vi "FPGA_Main_IX.vi"() -> ()   [LabVIEW 2018]
uses:
  <vilib>/LabVIEW Targets/FPGA/RIO/BlueMoonOnboardIO/nicrio_cRIO-BlueMoonOnboardAi_TerminalMod.ctl
  <vilib>/LabVIEW Targets/FPGA/RIO/BlueMoonOnboardIO/nicrio_cRIO-BlueMoonOnboardAi_VoltageRange.ctl
  <vilib>/Platform/TimedLoop/XDataNode/timing_clust.ctl
  <vilib>/Platform/TimedLoop/XDataNode/nitl_modes.ctl
  <vilib>/Platform/TimedLoop/XDataNode/wakeup.ctl
  ctl/_FPGA_priRFSettings_Parameters.ctl
  ctl/_FPGA_auxWfmSettings_Parameters.ctl
  <vilib>/rvi/Emulation/niFpgaGetClockAttributes.vi
  <vilib>/rvi/Emulation/niFpgaSctlEmulationGetInTimedLoop.vi
  <vilib>/rvi/Emulation/niFpgaEmulationReportErrorSimple.vi
  <vilib>/rvi/Emulation/niFpgaEmulationIsFPGAContextNoSignature.vi
  <vilib>/rvi/DataTransferAndStorage/Container/Common/niFpgaContainerGetUniqueNameForEmu.vi
  <vilib>/rvi/Memory/Memory_Emulation/niFpgaMemoryEmulationCacheClearOnFirstRun.vi
  <vilib>/rvi/Memory/Memory_Emulation/nirvimemoryEmulationManagerCache_MakeExclusive.vi
  <vilib>/rvi/Memory/Memory_Emulation/niFpgaMemoryEmulationValidateCache.vi
  <vilib>/rvi/Memory/Memory_Emulation/nirvimemoryEmulationManagerCache_InsertValue.vi
  <vilib>/Utility/error.llb/Clear Errors.vi
  <vilib>/rvi/Memory/Memory_Emulation/nirvimemoryEmulationManagerCache_ReleaseExclusive.vi
  <vilib>/rvi/Memory/Memory_Emulation/nirvimemoryEmulationManagerCache_GetValue.vi
  <vilib>/rvi/Memory/Memory_Emulation/nirvimemoryEmulationManagerCache_SetValue.vi
  <vilib>/rvi/Emulation/niFpgaProcessEmulError.vi
  <vilib>/rvi/eio/common/nirviEmuTemplateMethod_errors.vi
  <vilib>/rvi/Emulation/niFpgaCriticalErrorInLSC.vi
  <vilib>/rvi/eio/common/nirviEmuTemplatePropertySet_noerrors.vi
  <vilib>/rvi/errors/niFpgaSetErrorForExecOnDevCompSimple.vi
  <vilib>/rvi/eio/common/nirviEmuReportErrorAndStop.vi
  <vilib>/rvi/FIFO/Fifo_Resource/nirvififoEmulationSetSize.vi
  <vilib>/rvi/FIFO/Fifo_Resource/nirviFifoEmulationQueueMgr.vi
  <instcachedir>/0/nirviFifoEmulationQueueMgr_E5CAEC123FF24DC58D834DCA3CDAA9B5.lvgen/nirviFifoEmulationQueueMgr_E5CAEC123FF24DC58D834DCA3CDAA9B5_004.vi
  <vilib>/rvi/FIFO/Fifo_Resource/nirvififoEmulationDetermineInputValidOut.vi
  <vilib>/rvi/FIFO/Fifo_Resource/nirvififoEmulationCreateLock.vi
  <vilib>/rvi/FIFO/Fifo_Resource/nirvififoEmulationObtainLock.vi
  <vilib>/rvi/FIFO/Fifo_Resource/nirvififoEmulationReleaseLock.vi
  <vilib>/rvi/occurrence/nirviWaitOnOccurrenceBase.vi
  <vilib>/rvi/errors/nirviReportUnexpectedCaseInternalError.vi
  <vilib>/rvi/errors/nirviReportUnexpectedCaseInternalError (U32).vi
  <instcachedir>/0/nirviFifoEmulationQueueMgr_E5CAEC123FF24DC58D834DCA3CDAA9B5.lvgen/nirviFifoEmulationQueueMgr_E5CAEC123FF24DC58D834DCA3CDAA9B5_006.vi
  <instcachedir>/0/nirviFifoEmulationQueueMgr_E5CAEC123FF24DC58D834DCA3CDAA9B5.lvgen/nirviFifoEmulationQueueMgr_E5CAEC123FF24DC58D834DCA3CDAA9B5_002.vi
  <instrlib>/_niInstr/Basic Elements/v1/FPGA/Private/Count Down U16.vi
  <instrlib>/_niInstr/Basic Elements/v1/FPGA/Private/Count Down U32.vi
  <vilib>/rvi/interface/RandomDataEmulation/niFpgaRandomDataHandleErrors.vi
  <instcachedir>/0/nirviFifoEmulationQueueMgr_E5CAEC123FF24DC58D834DCA3CDAA9B5.lvgen/nirviFifoEmulationQueueMgr_E5CAEC123FF24DC58D834DCA3CDAA9B5_003.vi
  <vilib>/rvi/Memory/Memory_Emulation/nirvimemoryFastEmulation.vi
  <vilib>/rvi/Memory/Memory_Emulation/nirvimemoryEmulation.vi
  <vilib>/rvi/DataTransferAndStorage/Container/XNode/niFpgaContainer.xnode
  <vilib>/rvi/DataTransferAndStorage/Register/Emulation/niFpgaRegisterEmulation.vi
  <vilib>/eio/EIONode/EIONode.xnode
  <vilib>/eio/EIOPropertyNode/EIOPropertyNode.xnode
  <vilib>/rvi/FIFO/Fifo_Resource/nirvififoEmulationWrite.vi
  <vilib>/Platform/TimedLoop/XDataNode/XDataNode.xnode
  <vilib>/rvi/FIFO/Fifo_Resource/nirvififoEmulationRead.vi
  <vilib>/rvi/interface/RandomDataEmulation/nirviRandomDataFpgaReadWriteTemplate.vi
  <vilib>/rvi/FXPMathLib/FxpAdd/XNode/nifxpmath_Add.xnode
  <instrlib>/_niInstr/Basic Elements/v1/FPGA/niInstr Basic Elements v1 FPGA.lvlib
  <vilib>/rvi/FXPMathLib/sim/FxpSim.dll
  <vilib>/Platform/TimedLoop/XDataNode/XDNodeRunTimeDep.lvlib
  <vilib>/rvi/eio/common/nirviEmuTemplatePropertyGet_errors.vi
  <vilib>/rvi/eio/common/nirviEmuTemplatePropertyGet_noerrors.vi
  <vilib>/rvi/eio/common/nirviEmuTemplatePropertySet_errors.vi
panel:
  out "DI":u8
  out "Daq.AqNumber?":u32
  out "Daq.HighestValue_I16":i16
  out "Daq.Length?":u32
  out "Act.Timeout":u16
  out "Aux.Timeout":u16
  out "Pri.Timeout":u16
  out "AI.ReadingClocks":u32
  in  "Action":bool
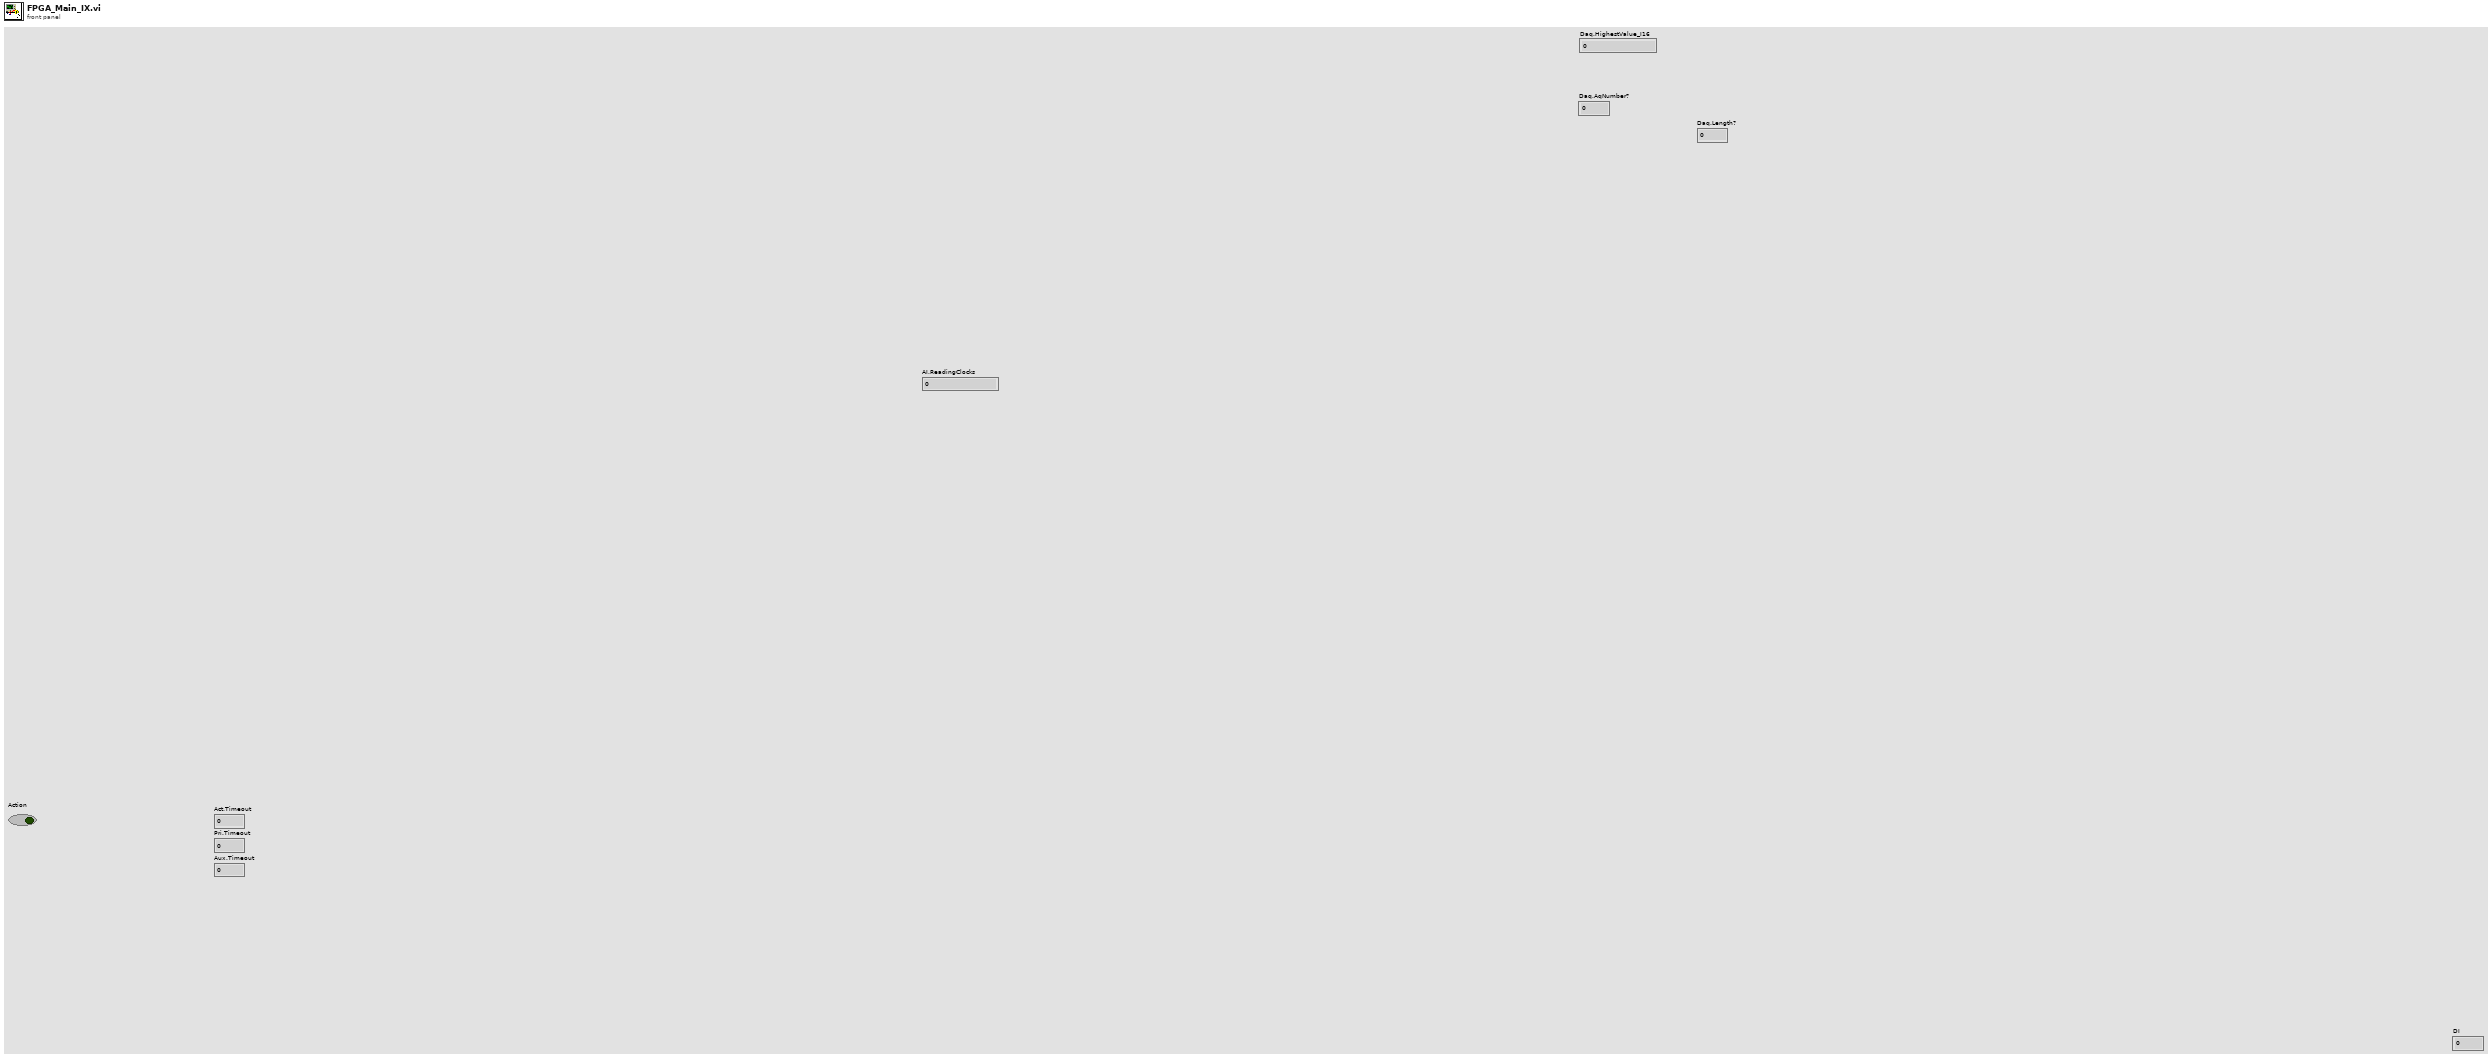
[diagram p1: front panel]
types:
  T1 = typedef "nicrio_cRIO-BlueMoonOnboardAi_VoltageRange.ctl" = u8
  T2 = typedef "nicrio_cRIO-BlueMoonOnboardAi_TerminalMod.ctl" = u8
  T3 = typedef "XDNodeRunTimeDep.lvlib/timing_clust.ctl" = cluster{"Expected End [f-1]":u64, "Actual End [f-1]":u64, "Finished Late? [f-1]":bool, "Expected End [i-1]":u64, "Actual End [i-1]":u64, "Finished Late? [i-1]":bool, "Expected Start [i]":u64, "Actual Start [i]":u64, "Expected Start [f]":u64, "Actual Start [f]":u64, "Source Name":string, "Structure Name":string, "Period":i64, "Deadline":i64, "Offset":i64, "Start":i64, "Priority":i32, "Timeout":i32, "Mode":T4, "Wakeup Reason":T5, "Error":errorcluster, "Source Type":string, "Secondary Source Type":string, "Global End Time":u64, "Global Start Time":u64, "Frame Duration":u64, "Iteration Duration":u64, "Assigned CPU":i32, "I/O Scan Engine Mode":u32}
  T4 = typedef "XDNodeRunTimeDep.lvlib/nitl_modes.ctl" = enum32{"No Change", "Process missed periods, maintain original phase", "Discard missed periods, maintain original phase", "Process missed periods, ignore original phase", "Discard missed periods, ignore original phase"}
  T5 = typedef "XDNodeRunTimeDep.lvlib/wakeup.ctl" = enum32{"Normal", "Aborted", "Asynchronous wakeup", "Timing source error", "Timed loop error", "Timeout"}
  T6 = typedef "_FPGA_auxWfmSettings_Parameters.ctl" = cluster{"PlsTicks":u16, "PlsInten":u16, "AuxBias":u16, "AuxTicks":u32, "Repeat":u32}
  T7 = typedef "_FPGA_priRFSettings_Parameters.ctl" = cluster{"CycleIncrement":u32, "Amp":u32, "Total Ticks":u32, "Conj Ticks":u16, "Repeat":u16}
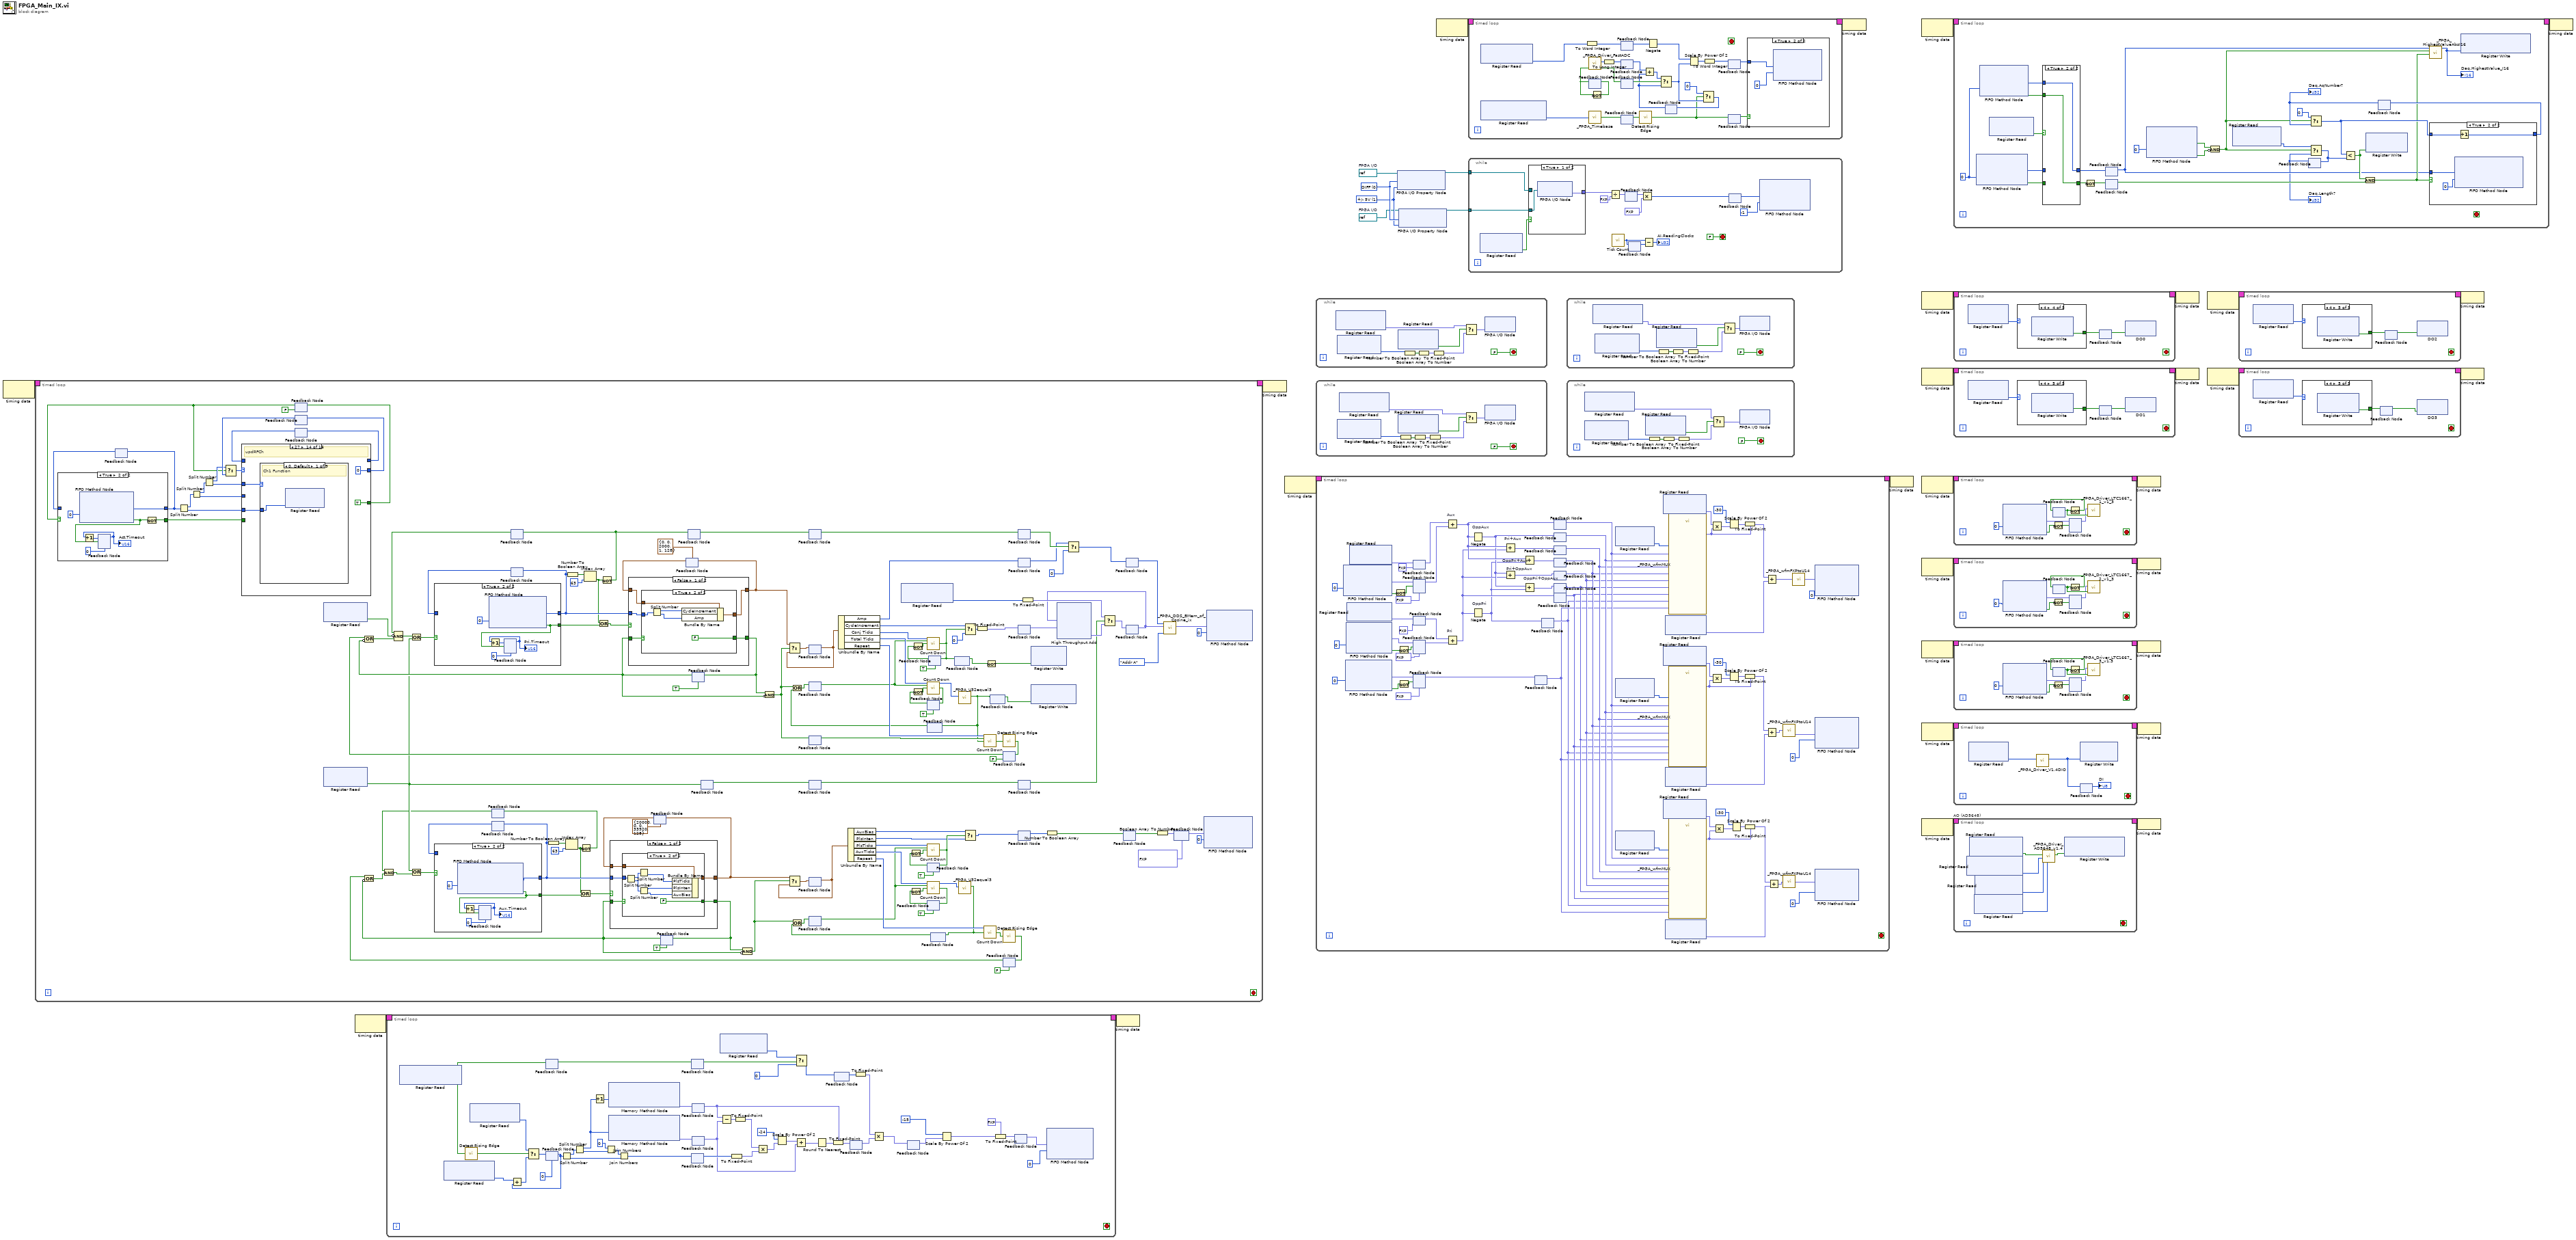
[diagram p0: block diagram]
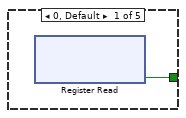
[diagram p2: hidden frame]
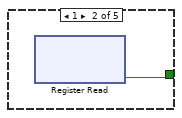
[diagram p3: hidden frame]
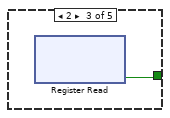
[diagram p4: hidden frame]
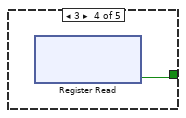
[diagram p5: hidden frame]
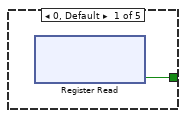
[diagram p6: hidden frame]
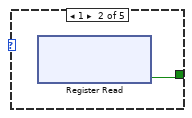
[diagram p7: hidden frame]
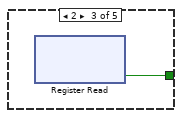
[diagram p8: hidden frame]
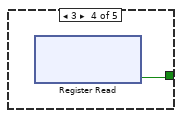
[diagram p9: hidden frame]
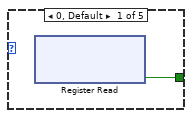
[diagram p10: hidden frame]
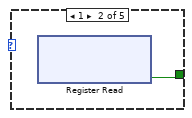
[diagram p11: hidden frame]
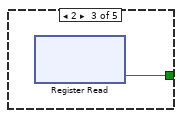
[diagram p12: hidden frame]
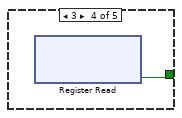
[diagram p13: hidden frame]
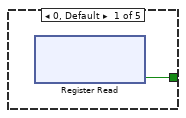
[diagram p14: hidden frame]
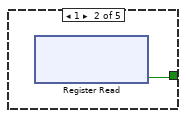
[diagram p15: hidden frame]
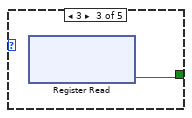
[diagram p16: hidden frame]
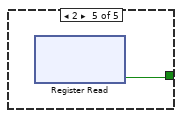
[diagram p17: hidden frame]
diagram:
  w22 = T1 1 items=["+/- 10V", "+/- 5V", "+/- 2V", "+/- 1V"] ("Voltage Range")
  w23 = T2 0 items=["DIFF", "RSE"] ("Terminal Mode")
  w19 = refnum<k21> "AI6"  # FPGA I/O
  w24 = refnum<k21> "AI7"  # FPGA I/O
  n1 = node-c288() -> (w32:T3)  [unwired: 1 in]
  n2 = timed-loop {
    timing: w32 -> [_]
    timing-out: [_] -> w31
    stop <- _ stop-if-true
    n3 = feedback #1() -> (w96:u64)  [unwired: 1 in]
    n4 = feedback #2(FALSE ("=1?")) -> (w40:bool)
    n5 = case shown="True" w40 {
      tunnel: [w234 w240] -> w95
      tunnel: w96 -> [w234 _]
      tunnel: [FALSE ("Timed Out?") w235] -> w94
      frame False {
      }
      frame True {
        n6 = xnode ("FIFO Method Node")("Timeout"=0) -> ("Element"=w240:u64, "Timed Out?"=w236:bool)  [unwired: 1 in, 1 out]
        n7 = feedback #3(u16 0) -> (w237:u16)
        "Act.Timeout" <- w237
        n8 = Increment(x=w237) -> (x+1=w238:u16)
        n9 = feedback-in #3(w238, w236) -> ()
        n10 = Not(x=w236) -> (.not. x?=w235:bool)
      }
    }
    n11 = feedback-in #1(w95) -> ()
    n12 = Split Number(x=w95) -> (hi(x)=w160:u32, lo(x)=w156:u32)
    n13 = Split Number(x=w160) -> (hi(x)=w159:u16, lo(x)=w157:u16)
    n14 = Split Number(x=w159) -> (hi(x)=w41:u8, lo(x)=w158:u8)
    n15 = feedback #4() -> (w173:u8)  [unwired: 1 in]
    n16 = Select(t=w41, s=w40, f=w173) -> (s? t:f=w42:u8)
    n17 = feedback #5() -> (w63:u32)  [unwired: 1 in]
    n18 = case shown="27" w42 {
      selector: w42 -> [w243 w244 w253 w257 w261 w264 w267 w277 w283 w288 _ w302 _ _ _ w350]
      tunnel: w158 -> [_ _ _ _ _ _ _ w276 _ _ w296 w308 _ w314 w344 _]
      tunnel: w157 -> [_ _ _ _ _ _ w270 _ _ _ w295 w307 _ _ _ _]
      tunnel: w156 -> [_ w251 w256 _ _ _ _ _ w279 _ _ w305 _ w313 w343 w352]
      tunnel: ["Action" w246 FALSE ("Timed Out?") TRUE ("Timed Out?") FALSE TRUE ("Timed Out?") TRUE TRUE TRUE ("Timed Out?") FALSE ("Timed Out?") TRUE ("Timed Out?") FALSE ("Timed Out?") TRUE ("Timed Out?") TRUE ("Timed Out?") TRUE ("Timed Out?") TRUE ("Timed Out?")] -> w155
      tunnel: w94 -> [_ w245 _ _ _ _ _ _ _ _ _ _ _ _ _ _]
      tunnel: [_ _ _ _ _ _ _ _ _ w284 _ _ _ _ _ w352] -> w64
      tunnel: w63 -> [_ _ _ _ _ _ _ _ _ _ w299 _ _ _ _ _]
      tunnel: [w243 w244 w252 w257 w260 w264 w267 w277 w283 w286 u8 0 w301 u8 0 u8 0 u8 0 w350] -> w43
      frame 0, Default {
        n19 = xnode ("Register Read")("Data"="Action") -> ()  [unwired: 1 in, 1 out]
      }
      frame 1 {
        # "Wait"
        n20 = feedback #6() -> (w249:bool)  [unwired: 1 in]
        n21 = call-poly <instrlib>:"Count Down.vi"("count in"=w251, "load"=w245, "decrement"=w249) -> ("count out"=w247:u32, "terminal count"=w248:bool)  [unwired: 11 in]
        n22 = Not(x=w248) -> (.not. x?=w250:bool)
        n23 = feedback-in #6(w250) -> ()
        n24 = call "_FPGA_U32equal1.vi"("Numeric"=w247) -> ("=1?"=w246:bool)  [unwired: 10 in]
      }
      frame 10 {
        # "DDS_Start..."
        n25 = xnode ("Register Write")("Data"=w256) -> ()  [unwired: 1 in, 1 out]
        n26 = xnode ("Register Write")("Data"=TRUE) -> ()  [unwired: 1 in, 1 out]
        n27 = Increment(x=w253) -> (x+1=w252:u8)
      }
      frame 11 {
        # "...DDS_Start"
        n28 = xnode ("Register Write")("Data"=FALSE) -> ()  [unwired: 1 in, 1 out]
      }
      frame 12 {
        # "DDS_Stop..."
        n29 = xnode ("Register Write")("Data"=TRUE) -> ()  [unwired: 1 in, 1 out]
        n30 = Increment(x=w261) -> (x+1=w260:u8)
      }
      frame 13 {
        # "...DDS_Stop"
        n31 = xnode ("Register Write")("Data"=FALSE) -> ()  [unwired: 1 in, 1 out]
      }
      frame 14 {
        # "DDS_UpdBias"
        n32 = Number To Boolean Array(number=w270) -> (Boolean array=w269:bool[])
        n33 = Boolean Array To Number(Boolean array=w269) -> (number=w268:fxp<+/-,16,14>)
        n34 = xnode ("Register Read")("Data"=w268) -> ()  [unwired: 1 in, 1 out]
      }
      frame 15 {
        # "Daq_Setup"
        n35 = Number To Boolean Array(number=w276) -> (Boolean array=w275:bool[])
        n36 = Index Array(array=w275, index #1=0 ("index")) -> (element #1=w272:bool, element #2=w273:bool)  [unwired: 1 in]
        n37 = xnode ("Register Read")("Data"=w272) -> ()  [unwired: 1 in, 1 out]
        n38 = xnode ("Register Read")("Data"=w273) -> ()  [unwired: 1 in, 1 out]
      }
      frame 16 {
        # "Daq_Start"
        n39 = xnode ("Register Read")("Data"=w279) -> ()  [unwired: 1 in, 1 out]
        n40 = xnode ("FIFO Method Node")("Element"=TRUE, "Timeout"=0) -> ()  [unwired: 1 in, 2 out]
      }
      frame 23 {
        # "updExtDO..."
        n41 = xnode ("Register Read")() -> ("Data"=w285:u8)  [unwired: 1 in, 1 out]
        n42 = Increment(x=w288) -> (x+1=w286:u8)
        n43 = To Unsigned Long Integer(number=w285) -> (unsigned 32bit integer=w284:u32)
      }
      frame 24 {
        # "...updExtDO"
        n44 = Number To Boolean Array(number=w295) -> (Boolean array=w294:bool[])
        n45 = To Unsigned Byte Integer(number=w299) -> (unsigned 8bit integer=w298:u8)
        n46 = Index Array(array=w294, index=0) -> (element=w292:bool)
        n47 = Number To Boolean Array(number=w298) -> (Boolean array=w297:bool[])
        n48 = Replace Array Subset(array=w297, new element=w292, index=w296) -> (w291:bool[])
        n49 = Boolean Array To Number(Boolean array=w291) -> (number=w290:u8)
        n50 = xnode ("Register Read")("Data"=w290) -> ()  [unwired: 1 in, 1 out]
      }
      frame 25 {
        # "updExtAO..."
        n51 = To Unsigned Byte Integer(number=w307) -> (unsigned 8bit integer=w306:u8)
        n52 = To Unsigned Word Integer(number=w305) -> (unsigned 16bit integer=w304:u16)
        n53 = Increment(x=w302) -> (x+1=w301:u8)
        n54 = xnode ("Register Read")("Data"=w308) -> ()  [unwired: 1 in, 1 out]
        n55 = xnode ("Register Read")("Data"=TRUE) -> ()  [unwired: 1 in, 1 out]
        n56 = xnode ("Register Read")("Data"=w306) -> ()  [unwired: 1 in, 1 out]
        n57 = xnode ("Register Read")("Data"=w304) -> ()  [unwired: 1 in, 1 out]
      }
      frame 26 {
        # "...updExtAO"
        n58 = xnode ("Register Read")("Data"=FALSE) -> ()  [unwired: 1 in, 1 out]
      }
      frame 27 {
        # "updRFCh"
        n59 = case shown="0, Default" w314 {
          tunnel: w313 -> [w317 w318 w319 w323 w327 w331 w333 w336 w339]
          frame 0, Default {
            # "Ch1 Function"
            n60 = xnode ("Register Read")("Data"=w317) -> ()  [unwired: 1 in, 1 out]
          }
          frame 1 {
            # "Ch2 Function"
            n61 = xnode ("Register Read")("Data"=w318) -> ()  [unwired: 1 in, 1 out]
          }
          frame 2 {
            # "Ch3 Function"
            n62 = xnode ("Register Read")("Data"=w319) -> ()  [unwired: 1 in, 1 out]
          }
          frame 3 {
            # "Ch1 Bias"
            n63 = Split Number(x=w323) -> (lo(x)=w322:u16)  [unwired: 1 out]
            n64 = Number To Boolean Array(number=w322) -> (Boolean array=w321:bool[])
            n65 = Boolean Array To Number(Boolean array=w321) -> (number=w320:fxp<+/-,16,14>)
            n66 = xnode ("Register Read")("Data"=w320) -> ()  [unwired: 1 in, 1 out]
          }
          frame 4 {
            # "Ch2 Bias"
            n67 = Split Number(x=w327) -> (lo(x)=w326:u16)  [unwired: 1 out]
            n68 = Number To Boolean Array(number=w326) -> (Boolean array=w325:bool[])
            n69 = Boolean Array To Number(Boolean array=w325) -> (number=w324:fxp<+/-,16,14>)
            n70 = xnode ("Register Read")("Data"=w324) -> ()  [unwired: 1 in, 1 out]
          }
          frame 5 {
            # "Ch3 Bias"
            n71 = Split Number(x=w331) -> (lo(x)=w330:u16)  [unwired: 1 out]
            n72 = Number To Boolean Array(number=w330) -> (Boolean array=w329:bool[])
            n73 = Boolean Array To Number(Boolean array=w329) -> (number=w328:fxp<+/-,16,14>)
            n74 = xnode ("Register Read")("Data"=w328) -> ()  [unwired: 1 in, 1 out]
          }
          frame 6 {
            # "Ch1 Scale"
            n75 = Number To Boolean Array(number=w333) -> (Boolean array=w334:bool[])
            n76 = Boolean Array To Number(Boolean array=w334) -> (number=w332:fxp<+,32,32>)
            n77 = xnode ("Register Read")("Data"=w332) -> ()  [unwired: 1 in, 1 out]
          }
          frame 7 {
            # "Ch2 Scale"
            n78 = Number To Boolean Array(number=w336) -> (Boolean array=w337:bool[])
            n79 = Boolean Array To Number(Boolean array=w337) -> (number=w335:fxp<+,32,32>)
            n80 = xnode ("Register Read")("Data"=w335) -> ()  [unwired: 1 in, 1 out]
          }
          frame 8 {
            # "Ch2 Scale"
            n81 = Number To Boolean Array(number=w339) -> (Boolean array=w340:bool[])
            n82 = Boolean Array To Number(Boolean array=w340) -> (number=w338:fxp<+,32,32>)
            n83 = xnode ("Register Read")("Data"=w338) -> ()  [unwired: 1 in, 1 out]
          }
        }
      }
      frame 200 {
        # "FGEN"
        n84 = case shown="4" w344 {
          tunnel: w343 -> [w345 w346 w347 _ _]
          frame 0, Default {
            n85 = xnode ("Register Write")("Data"=w345) -> ()  [unwired: 1 in, 1 out]
          }
          frame 1 {
            n86 = xnode ("Register Write")("Data"=w346) -> ()  [unwired: 1 in, 1 out]
          }
          frame 2 {
            n87 = xnode ("Register Write")("Data"=w347) -> ()  [unwired: 1 in, 1 out]
          }
          frame 3 {
            # "Start"
            n88 = xnode ("Register Write")("Data"=TRUE) -> ()  [unwired: 1 in, 1 out]
          }
          frame 4 {
            # "Stop"
            n89 = xnode ("Register Write")("Data"=FALSE) -> ()  [unwired: 1 in, 1 out]
          }
        }
      }
      frame 255 {
      }
    }
    n90 = feedback-in #2(w155) -> ()
    n91 = feedback-in #4(w43) -> ()
    n92 = feedback-in #5(w64) -> ()
    n93 = xnode ("Register Read")() -> ("Data"=w45:bool)  [unwired: 1 in, 1 out]
    n94 = xnode ("Register Read")() -> ("Data"=w73:bool)  [unwired: 1 in, 1 out]
    n95 = feedback #7() -> (w70:bool)  [unwired: 1 in]
    n96 = feedback #8() -> (w118:u64)  [unwired: 1 in]
    n97 = feedback #9() -> (w89:bool)  [unwired: 1 in]
    n98 = feedback #10() -> (w123:u64)  [unwired: 1 in]
    n99 = feedback #11(T6 {"PlsTicks"=20000, "PlsInten"=0, "AuxBias"=0, "AuxTicks"=33920, "Repeat"=128} ("Cluster")) -> (w149:T6)
    n100 = feedback #12(TRUE) -> (w66:bool)
    n101 = feedback #13(T7 {"CycleIncrement"=0, "Amp"=0, "Total Ticks"=2000, "Conj Ticks"=1, "Repeat"=128} ("RF Set")) -> (w152:T7)
    n102 = feedback #14() -> (w86:bool)  [unwired: 1 in]
    n103 = feedback #15(TRUE) -> (w121:bool)
    n104 = feedback-in #16(w73) -> ()
    n105 = feedback #16() -> (w87:bool)  [unwired: 1 in]
    n106 = feedback #17() -> (w85:bool)  [unwired: 1 in]
    n107 = feedback-in #17(w86) -> ()
    n108 = feedback #18() -> (w143:T7)  [unwired: 1 in]
    n109 = feedback #19() -> (w59:bool)  [unwired: 1 in]
    n110 = feedback #20() -> (w134:bool)  [unwired: 1 in]
    n111 = feedback-in #21(w87) -> ()
    n112 = feedback #21() -> (w128:bool)  [unwired: 1 in]
    n113 = feedback #22() -> (w117:T6)  [unwired: 1 in]
    n114 = feedback #23() -> (w54:bool)  [unwired: 1 in]
    n115 = Unbundle By Name(w143) -> ("Amp"=w161:u32, "CycleIncrement"=w164:u32, "Conj Ticks"=w172:u16, "Total Ticks"=w162:u32, "Repeat"=w137:u16)
    n116 = Unbundle By Name(w117) -> ("AuxBias"=w104:u16, "PlsInten"=w103:u16, "PlsTicks"=w116:u16, "AuxTicks"=w108:u32, "Repeat"=w106:u32)
    n117 = xnode ("Register Read")() -> ("Data"=w139:u32)  [unwired: 1 in, 1 out]
    n118 = feedback #24(TRUE ("terminal count")) -> (w166:bool)
    n119 = Not(x=w166) -> (.not. x?=w165:bool)
    n120 = call-poly <instrlib>:"Count Down.vi"("count in"=w162, "load"=w59, "decrement"=w165) -> ("count out"=w120:u32, "terminal count"=w167:bool)  [unwired: 11 in]
    n121 = feedback-in #24(w167) -> ()
    n122 = feedback #25() -> (w62:bool)  [unwired: 1 in]
    n123 = feedback #26(TRUE ("terminal count")) -> (w113:bool)
    n124 = Not(x=w113) -> (.not. x?=w114:bool)
    n125 = call-poly <instrlib>:"Count Down.vi"("count in"=w116, "load"=w54, "decrement"=w114) -> ("terminal count"=w105:bool)  [unwired: 11 in, 1 out]
    n126 = feedback-in #26(w105) -> ()
    n127 = feedback #27(TRUE ("terminal count")) -> (w111:bool)
    n128 = Not(x=w111) -> (.not. x?=w110:bool)
    n129 = call-poly <instrlib>:"Count Down.vi"("count in"=w108, "load"=w54, "decrement"=w110) -> ("count out"=w102:u32, "terminal count"=w112:bool)  [unwired: 11 in]
    n130 = feedback-in #27(w112) -> ()
    n131 = feedback #28(TRUE ("terminal count")) -> (w170:bool)
    n132 = Not(x=w170) -> (.not. x?=w169:bool)
    n133 = call-poly <instrlib>:"Count Down.vi"("count in"=w172, "load"=w59, "decrement"=w169) -> ("terminal count"=w39:bool)  [unwired: 11 in, 1 out]
    n134 = feedback-in #28(w39) -> ()
    n135 = feedback #29() -> (w56:bool)  [unwired: 1 in]
    n136 = feedback #30() -> (w38:bool)  [unwired: 1 in]
    n137 = feedback-in #30(w39) -> ()
    n138 = call "_FPGA_U32equal3.vi"("Numeric"=w120) -> ("==3?"=w36:bool)  [unwired: 10 in]
    n139 = feedback-in #25(w36) -> ()
    n140 = call "_FPGA_U32equal3.vi"("Numeric"=w102) -> ("==3?"=w57:bool)  [unwired: 10 in]
    n141 = feedback-in #29(w57) -> ()
    n142 = Select(t=w164, s=w39, f=u32 0) -> (s? t:f=w146:u32)
    n143 = Select(t=w104, s=w105, f=w103) -> (s? t:f=w53:u16)
    n144 = To Fixed-Point(number=w146) -> (fixed-point=w145:fxp<+,32,32>)  [unwired: 1 in]
    n145 = call-poly <instrlib>:"Count Down.vi"("count in"=w137, "load"=w134, "decrement"=w36) -> ("terminal count"=w136:bool)  [unwired: 11 in, 1 out]
    n146 = call-poly <instrlib>:"Count Down.vi"("count in"=w106, "decrement"=w57) -> ("terminal count"=w101:bool)  [unwired: 12 in, 1 out]
    n147 = Not(x=w38) -> (.not. x?=w37:bool)
    n148 = feedback #31() -> (w35:bool)  [unwired: 1 in]
    n149 = feedback-in #31(w36) -> ()
    n150 = call <instrlib>:"Detect Rising Edge.vi"("signal"=w136) -> ("edge detected"=w135:bool)  [unwired: 14 in]
    n151 = feedback #32(FALSE ("edge detected")) -> (w91:bool)
    n152 = Compound Arithmetic op=OR(w91, invert w121) -> (w44:bool)
    n153 = Compound Arithmetic op=AND(w89, invert w45, w44) -> (w90:bool)
    n154 = Or(x=w90, y=w73) -> (x .or. y?=w88:bool)
    n155 = case shown="True" w88 {
      tunnel: [w204 w211] -> w93
      tunnel: [TRUE ("Timed Out?") w209] -> w99
      tunnel: w123 -> [w204 _]
      frame False {
      }
      frame True {
        n156 = xnode ("FIFO Method Node")("Timeout"=0) -> ("Element"=w211:u64, "Timed Out?"=w209:bool)  [unwired: 1 in, 1 out]
        n157 = feedback #33(u16 0) -> (w206:u16)
        "Pri.Timeout" <- w206
        n158 = Increment(x=w206) -> (x+1=w207:u16)
        n159 = feedback-in #33(w207, w209) -> ()
      }
    }
    n160 = feedback-in #10(w93) -> ()
    n161 = Number To Boolean Array(number=w93) -> (Boolean array=w98:bool[])
    n162 = Index Array(array=w98, index=63) -> (element=w83:bool)
    n163 = Or(x=w83, y=w99) -> (x .or. y?=w92:bool)
    n164 = Not(x=w83) -> (.not. x?=w81:bool)
    n165 = feedback-in #9(w81) -> ()
    n166 = case shown="False" w92 {
      tunnel: w152 -> [w216 w231]
      tunnel: w93 -> [w215 _]
      tunnel: [w214 w231] -> w151
      tunnel: [w213 w232] -> w122
      tunnel: w121 -> [w212 w232]
      frame False {
        n167 = case shown="True" w212 {
          tunnel: w216 -> [w224 w230]
          tunnel: w215 -> [w223 w229]
          tunnel: [w221 w226] -> w214
          tunnel: [TRUE FALSE] -> w213
          frame False {
            n168 = Split Number(x=w223) -> (hi(x)=w222:u32, lo(x)=w219:u32)
            n169 = Split Number(x=w219) -> (hi(x)=w218:u16, lo(x)=w217:u16)
            n170 = Bundle By Name(cluster=w224, "Total Ticks"=w222, "Conj Ticks"=w218, "Repeat"=w217) -> (w221:T7)
          }
          frame True {
            n171 = Split Number(x=w229) -> (hi(x)=w228:u32, lo(x)=w227:u32)
            n172 = Bundle By Name(cluster=w230, "CycleIncrement"=w228, "Amp"=w227) -> (w226:T7)
          }
        }
      }
      frame True {
      }
    }
    n173 = feedback-in #13(w151) -> ()
    n174 = feedback-in #14(w81) -> ()
    n175 = feedback-in #15(w122) -> ()
    n176 = Compound Arithmetic op=AND(w122, invert w121) -> (w61:bool)
    n177 = Select(t=w151, s=w61, f=w143) -> (s? t:f=w150:T7)
    n178 = Or(x=w61, y=w62) -> (x .or. y?=w60:bool)
    n179 = feedback-in #18(w150) -> ()
    n180 = feedback-in #19(w60) -> ()
    n181 = feedback-in #20(w61) -> ()
    n182 = feedback-in #32(w135) -> ()
    n183 = call <instrlib>:"Detect Rising Edge.vi"("signal"=w101) -> ("edge detected"=w100:bool)  [unwired: 14 in]
    n184 = feedback #34(FALSE ("terminal count")) -> (w65:bool)
    n185 = Compound Arithmetic op=OR(w65, invert w66) -> (w68:bool)
    n186 = And(x=w70, y=w68) -> (x .and. y?=w69:bool)
    n187 = Or(x=w73, y=w69) -> (x .or. y?=w72:bool)
    n188 = case shown="True" w72 {
      tunnel: [w175 w181] -> w76
      tunnel: [TRUE ("Timed Out?") w176] -> w119
      tunnel: w118 -> [w175 _]
      frame False {
      }
      frame True {
        n189 = xnode ("FIFO Method Node")("Timeout"=0) -> ("Element"=w181:u64, "Timed Out?"=w176:bool)  [unwired: 1 in, 1 out]
        n190 = feedback #35(u16 0) -> (w177:u16)
        "Aux.Timeout" <- w177
        n191 = Increment(x=w177) -> (x+1=w178:u16)
        n192 = feedback-in #35(w178, w176) -> ()
      }
    }
    n193 = feedback-in #8(w76) -> ()
    n194 = Number To Boolean Array(number=w76) -> (Boolean array=w77:bool[])
    n195 = Index Array(array=w77, index=63) -> (element=w74:bool)
    n196 = Or(x=w74, y=w119) -> (x .or. y?=w75:bool)
    n197 = Not(x=w74) -> (.not. x?=w71:bool)
    n198 = feedback-in #7(w71) -> ()
    n199 = case shown="False" w75 {
      tunnel: w149 -> [w186 w202]
      tunnel: w76 -> [w185 _]
      tunnel: [w184 w202] -> w125
      tunnel: [w183 w203] -> w67
      tunnel: w66 -> [w182 w203]
      frame False {
        n200 = case shown="True" w182 {
          tunnel: w186 -> [w192 w201]
          tunnel: w185 -> [w191 w200]
          tunnel: [w189 w199] -> w184
          tunnel: [TRUE FALSE] -> w183
          frame False {
            n201 = Split Number(x=w191) -> (hi(x)=w190:u32, lo(x)=w187:u32)
            n202 = Bundle By Name(cluster=w192, "AuxTicks"=w190, "Repeat"=w187) -> (w189:T6)
          }
          frame True {
            n203 = Split Number(x=w200) -> (hi(x)=w197:u32, lo(x)=w196:u32)
            n204 = Split Number(x=w197) -> (lo(x)=w195:u16)  [unwired: 1 out]
            n205 = Split Number(x=w196) -> (hi(x)=w194:u16, lo(x)=w193:u16)
            n206 = Bundle By Name(cluster=w201, "PlsTicks"=w195, "PlsInten"=w194, "AuxBias"=w193) -> (w199:T6)
          }
        }
      }
      frame True {
      }
    }
    n207 = feedback-in #11(w125) -> ()
    n208 = feedback-in #12(w67) -> ()
    n209 = Compound Arithmetic op=AND(w67, invert w66) -> (w55:bool)
    n210 = Select(t=w125, s=w55, f=w117) -> (s? t:f=w126:T6)
    n211 = Or(x=w55, y=w56) -> (x .or. y?=w58:bool)
    n212 = feedback-in #22(w126) -> ()
    n213 = feedback-in #23(w58) -> ()
    n214 = feedback-in #34(w100) -> ()
    n215 = feedback #36() -> (w84:bool)  [unwired: 1 in]
    n216 = feedback-in #36(w85) -> ()
    n217 = feedback #37() -> (w80:u32)  [unwired: 1 in]
    n218 = feedback-in #37(w161) -> ()
    n219 = feedback #38() -> (w144:fxp<+,32,32>)  [unwired: 1 in]
    n220 = feedback-in #38(w145) -> ()
    n221 = feedback #39() -> (w140:bool)  [unwired: 1 in]
    n222 = feedback-in #39(w128) -> ()
    n223 = feedback #40() -> (w52:u16)  [unwired: 1 in]
    n224 = feedback-in #40(w53) -> ()
    n225 = To Fixed-Point(number=w139) -> (fixed-point=w138:fxp<+,32,32>)  [unwired: 1 in]
    n226 = xnode ("Register Write")("Data"=w37) -> ()  [unwired: 1 in, 1 out]
    n227 = xnode ("Register Write")("Data"=w35) -> ()  [unwired: 1 in, 1 out]
    n228 = Number To Boolean Array(number=w52) -> (Boolean array=w51:bool[])
    n229 = Select(t=w80, s=w84, f=u32 0 ("t")) -> (s? t:f=w82:u32)
    n230 = feedback #41() -> (w50:bool[])  [unwired: 1 in]
    n231 = feedback-in #41(w51) -> ()
    n232 = feedback #42() -> (w132:u32)  [unwired: 1 in]
    n233 = feedback-in #42(w82) -> ()
    n234 = feedback #43() -> (w133:fxp<+,32,32>)  [unwired: 1 in]
    n235 = xnode ("High Throughput Add")("x"=w133, "y"=w144) -> ("x+y"=w141:fxp<+,32,32>)
    n236 = Select(t=w138, s=w140, f=w141) -> (s? t:f=w142:fxp<+,32,32>)
    n237 = feedback-in #43(w142) -> ()
    n238 = Boolean Array To Number(Boolean array=w50) -> (number=w49:fxp<+/-,16,14>)
    n239 = call "_FPGA_DDS_BMem_of_Cosine_ix.vi"("Addr"=enum16{"Addr A", "Addr B"}."Addr A", "Cycle_in"=w133, "NormAmp*2^29"=w132) -> ("A x COS"=w129:fxp<+/-,16,14>)  [unwired: 8 in]
    n240 = feedback #44(fxp<+/-,16,14>[] [8191.5, 8191.5]) -> (w48:fxp<+/-,16,14>)
    n241 = feedback-in #44(w49) -> ()
    n242 = xnode ("FIFO Method Node")("Element"=w48, "Timeout"=0) -> ()  [unwired: 1 in, 2 out]
    n243 = xnode ("FIFO Method Node")("Element"=w129, "Timeout"=0) -> ()  [unwired: 1 in, 2 out]
  }
  n244 = node-c288() -> (w2:T3)  [unwired: 1 in]
  n245 = timed-loop {
    timing: w2 -> [_]
    timing-out: [_] -> w1
    stop <- _ stop-if-true
    n246 = xnode ("Register Read")() -> ("Data"=w355:bool)  [unwired: 1 in, 1 out]
    n247 = xnode ("Register Read")() -> ("Data"=w397:u32)  [unwired: 1 in, 1 out]
    n248 = call <instrlib>:"Detect Rising Edge.vi"("signal"=w355) -> ("edge detected"=w356:bool)  [unwired: 14 in]
    n249 = xnode ("Register Read")() -> ("Data"=w362:u32)  [unwired: 1 in, 1 out]
    n250 = feedback-in #45(w355) -> ()
    n251 = feedback #45() -> (w359:bool)  [unwired: 1 in]
    n252 = feedback #46(u32 0) -> (w394:u32)
    n253 = Add(x=w397, y=w394) -> (x+y=w363:u32)
    n254 = Select(t=w362, s=w356, f=w363) -> (s? t:f=w364:u32)
    n255 = feedback-in #46(w364) -> ()
    n256 = Split Number(x=w394) -> (hi(x)=w399:u16, lo(x)=w389:u16)
    n257 = Split Number(x=w399) -> (hi(x)=w393:u8, lo(x)=w392:u8)
    n258 = Increment(x=w393) -> (x+1=w398:u8)
    n259 = Join Numbers(hi=u8 0, lo=w392) -> ((hi.lo)=w390:u16)
    n260 = xnode ("Memory Method Node")("Address A"=w398) -> ("Data A"=w396:fxp<+/-,28,14>)  [unwired: 1 in, 1 out]
    n261 = xnode ("Memory Method Node")("Address B"=w393) -> ("Data B"=w395:fxp<+/-,28,14>)  [unwired: 1 in, 1 out]
    n262 = Join Numbers(hi=w390, lo=w389) -> ((hi.lo)=w388:u32)
    n263 = feedback #47() -> (w358:bool)  [unwired: 1 in]
    n264 = feedback-in #47(w359) -> ()
    n265 = feedback-in #48(w388) -> ()
    n266 = feedback #48() -> (w379:u32)  [unwired: 1 in]
    n267 = feedback-in #49(w396) -> ()
    n268 = feedback #49() -> (w376:fxp<+/-,28,14>)  [unwired: 1 in]
    n269 = feedback-in #50(w395) -> ()
    n270 = feedback #50() -> (w369:fxp<+/-,28,14>)  [unwired: 1 in]
    n271 = xnode ("Register Read")() -> ("Data"=w361:u16)  [unwired: 1 in, 1 out]
    n272 = Subtract(x=w376, y=w369) -> (x-y=w378:fxp<+/-,29,15>)
    n273 = To Fixed-Point(number=w379) -> (fixed-point=w387:fxp<+,24,24>)  [unwired: 1 in]
    n274 = To Fixed-Point(number=w378) -> (fixed-point=w377:fxp<+/-,23,9>)  [unwired: 1 in]
    n275 = Multiply(x=w377, y=w387) -> (x*y=w386:fxp<+/-,47,33>)
    n276 = Scale By Power Of 2(n=i16 -24, x=w386) -> (x*2^n=w384:fxp<+/-,47,33>)
    n277 = Select(t=w361, s=w358, f=u16 0) -> (s? t:f=w360:u16)
    n278 = Add(x=w384, y=w369) -> (x+y=w380:fxp<+/-,48,34>)
    n279 = Round To Nearest(number=w380) -> (nearest integer value=w383:fxp<+/-,34,34>)
    n280 = To Fixed-Point(fixed-point type=w376, number=w383) -> (fixed-point=w382:fxp<+/-,28,14>)
    n281 = feedback-in #51(w360) -> ()
    n282 = feedback #51() -> (w374:u16)  [unwired: 1 in]
    n283 = feedback-in #52(w382) -> ()
    n284 = feedback #52() -> (w375:fxp<+/-,28,14>)  [unwired: 1 in]
    n285 = To Fixed-Point(number=w374) -> (fixed-point=w373:fxp<+,32,32>)  [unwired: 1 in]
    n286 = Multiply(x=w373, y=w375) -> (x*y=w372:fxp<+/-,60,46>)
    n287 = feedback-in #53(w372) -> ()
    n288 = feedback #53() -> (w371:fxp<+/-,60,46>)  [unwired: 1 in]
    n289 = Scale By Power Of 2(n=i16 -15, x=w371) -> (x*2^n=w365:fxp<+/-,60,46>)
    n290 = To Fixed-Point(fixed-point type=fxp<+/-,16,14> 0.0 ("Element"), number=w365) -> (fixed-point=w367:fxp<+/-,16,14>)
    n291 = feedback #54() -> (w366:fxp<+/-,16,14>)  [unwired: 1 in]
    n292 = feedback-in #54(w367) -> ()
    n293 = xnode ("FIFO Method Node")("Element"=w366, "Timeout"=0) -> ()  [unwired: 1 in, 2 out]
  }
  n294 = node-c288(w1) -> ()
  n295 = node-c288(w31) -> ()
  n296 = node-c288() -> (w34:T3)  [unwired: 1 in]
  n297 = while {
    stop <- FALSE stop-if-true
    n298 = xnode ("Register Read")() -> ("Data"=w409:fxp<+/-,20,5>)  [unwired: 1 in, 1 out]
    n299 = xnode ("Register Read")() -> ("Data"=w405:u32)  [unwired: 1 in, 1 out]
    n300 = xnode ("Register Read")() -> ("Data"=w408:bool)  [unwired: 1 in, 1 out]
    n301 = Number To Boolean Array(number=w405) -> (Boolean array=w406:bool[])
    n302 = Boolean Array To Number(Boolean array=w406) -> (number=w407:fxp<+/-,32,5>)
    n303 = To Fixed-Point(number=w407) -> (fixed-point=w404:fxp<+/-,20,5>)  [unwired: 1 in]
    n304 = Select(t=w409, s=w408, f=w404) -> (s? t:f=w410:fxp<+/-,20,5>)
    n305 = xnode "FPGA I/O Node"("AO0"=w410) -> ()  [unwired: 1 in, 1 out]
  }
  n306 = while {
    stop <- FALSE stop-if-true
    n307 = xnode ("Register Read")() -> ("Data"=w417:u32)  [unwired: 1 in, 1 out]
    n308 = xnode ("Register Read")() -> ("Data"=w412:fxp<+/-,20,5>)  [unwired: 1 in, 1 out]
    n309 = xnode ("Register Read")() -> ("Data"=w414:bool)  [unwired: 1 in, 1 out]
    n310 = Number To Boolean Array(number=w417) -> (Boolean array=w415:bool[])
    n311 = Boolean Array To Number(Boolean array=w415) -> (number=w416:fxp<+/-,32,5>)
    n312 = To Fixed-Point(number=w416) -> (fixed-point=w418:fxp<+/-,20,5>)  [unwired: 1 in]
    n313 = Select(t=w412, s=w414, f=w418) -> (s? t:f=w413:fxp<+/-,20,5>)
    n314 = xnode "FPGA I/O Node"("AO1"=w413) -> ()  [unwired: 1 in, 1 out]
  }
  n315 = timed-loop {
    timing: w34 -> [_]
    timing-out: [_] -> w33
    stop <- _ stop-if-true
    n316 = xnode ("FIFO Method Node")("Timeout"=0) -> ("Element"=w490:fxp<+/-,16,14>, "Timed Out?"=w492:bool)  [unwired: 1 in, 1 out]
    n317 = xnode ("FIFO Method Node")("Timeout"=0) -> ("Element"=w485:fxp<+/-,16,14>, "Timed Out?"=w484:bool)  [unwired: 1 in, 1 out]
    n318 = xnode ("FIFO Method Node")("Timeout"=0) -> ("Element"=w488:fxp<+/-,16,14>, "Timed Out?"=w487:bool)  [unwired: 1 in, 1 out]
    n319 = xnode ("Register Read")() -> ("Data"=w481:fxp<+/-,16,14>)  [unwired: 1 in, 1 out]
    n320 = xnode ("Register Read")() -> ("Data"=w482:fxp<+/-,16,14>)  [unwired: 1 in, 1 out]
    n321 = Not(x=w492) -> (.not. x?=w491:bool)
    n322 = Not(x=w487) -> (.not. x?=w489:bool)
    n323 = Not(x=w484) -> (.not. x?=w486:bool)
    n324 = feedback-in #55(w482) -> ()
    n325 = feedback #55(fxp<+/-,16,14> 0.0 ("Data")) -> (w479:fxp<+/-,16,14>)
    n326 = feedback #56(fxp<+/-,16,14> 8191.5 ("Element")) -> (w480:fxp<+/-,16,14>)
    n327 = feedback-in #56(w490, w491) -> ()
    n328 = feedback #57(fxp<+/-,16,14> 0.0 ("Data")) -> (w478:fxp<+/-,16,14>)
    n329 = feedback-in #57(w481) -> ()
    n330 = feedback #58(fxp<+/-,16,14> 8191.5 ("Element")) -> (w477:fxp<+/-,16,14>)
    n331 = feedback-in #58(w488, w489) -> ()
    n332 = feedback #59(fxp<+/-,16,14> 8191.5 ("Element")) -> (w419:fxp<+/-,16,14>)
    n333 = feedback-in #59(w485, w486) -> ()
    n334 = Add "Aux"(x=w479, y=w480) -> (x+y=w436:fxp<+/-,16,14>)
    n335 = Add "Pri"(x=w478, y=w477) -> (x+y=w423:fxp<+/-,16,14>)
    n336 = Negate "OppAux"(x=w436) -> (-x=w434:fxp<+/-,16,14>)
    n337 = Negate "OppPri"(x=w423) -> (-x=w422:fxp<+/-,16,14>)
    n338 = Add "Pri+Aux"(x=w436, y=w423) -> (x+y=w432:fxp<+/-,16,14>)
    n339 = Add "Pri+OppAux"(x=w434, y=w423) -> (x+y=w428:fxp<+/-,16,14>)
    n340 = Add "OppPri+Aux"(x=w436, y=w422) -> (x+y=w430:fxp<+/-,16,14>)
    n341 = Add "OppPri+OppAux"(x=w434, y=w422) -> (x+y=w425:fxp<+/-,16,14>)
    n342 = feedback #60() -> (w420:fxp<+/-,16,14>)  [unwired: 1 in]
    n343 = feedback-in #60(w419) -> ()
    n344 = feedback #61() -> (w421:fxp<+/-,16,14>)  [unwired: 1 in]
    n345 = feedback-in #61(w422) -> ()
    n346 = feedback-in #62(w436) -> ()
    n347 = feedback #62() -> (w435:fxp<+/-,16,14>)  [unwired: 1 in]
    n348 = feedback #63() -> (w433:fxp<+/-,16,14>)  [unwired: 1 in]
    n349 = feedback-in #63(w434) -> ()
    n350 = feedback #64() -> (w431:fxp<+/-,16,14>)  [unwired: 1 in]
    n351 = feedback-in #64(w432) -> ()
    n352 = feedback #65() -> (w429:fxp<+/-,16,14>)  [unwired: 1 in]
    n353 = feedback-in #65(w430) -> ()
    n354 = feedback #66() -> (w427:fxp<+/-,16,14>)  [unwired: 1 in]
    n355 = feedback-in #66(w428) -> ()
    n356 = feedback #67() -> (w426:fxp<+/-,16,14>)  [unwired: 1 in]
    n357 = feedback-in #67(w425) -> ()
    n358 = feedback #68() -> (w424:fxp<+/-,16,14>)  [unwired: 1 in]
    n359 = feedback-in #68(w423) -> ()
    n360 = xnode ("Register Read")() -> ("Data"=w473:u8)  [unwired: 1 in, 1 out]
    n361 = xnode ("Register Read")() -> ("Data"=w468:u8)  [unwired: 1 in, 1 out]
    n362 = xnode ("Register Read")() -> ("Data"=w463:u8)  [unwired: 1 in, 1 out]
    n363 = xnode ("Register Read")() -> ("Data"=w452:fxp<+,32,32>)  [unwired: 1 in, 1 out]
    n364 = xnode ("Register Read")() -> ("Data"=w458:fxp<+,32,32>)  [unwired: 1 in, 1 out]
    n365 = xnode ("Register Read")() -> ("Data"=w446:fxp<+,32,32>)  [unwired: 1 in, 1 out]
    n366 = xnode ("Register Read")() -> ("Data"=w475:fxp<+/-,16,14>)  [unwired: 1 in, 1 out]
    n367 = xnode ("Register Read")() -> ("Data"=w470:fxp<+/-,16,14>)  [unwired: 1 in, 1 out]
    n368 = xnode ("Register Read")() -> ("Data"=w465:fxp<+/-,16,14>)  [unwired: 1 in, 1 out]
    n369 = call "_FPGA_wfmMUX.vi"("OppAux"=w433, "Aux"=w435, "Sel"=w473, "OppPri"=w421, "Pri+Aux"=w431, "OppPri+OppAux"=w426, "FGEN"=w420, "Pri+OppAux"=w427, "OppPri+Aux"=w429, "Pri"=w424) -> ("SelectedWfm"=w450:fxp<+/-,16,14>)  [unwired: 5 in]
    n370 = call "_FPGA_wfmMUX.vi"("OppAux"=w433, "Aux"=w435, "Sel"=w468, "OppPri"=w421, "Pri+Aux"=w431, "OppPri+OppAux"=w426, "FGEN"=w420, "Pri+OppAux"=w427, "OppPri+Aux"=w429, "Pri"=w424) -> ("SelectedWfm"=w456:fxp<+/-,16,14>)  [unwired: 5 in]
    n371 = call "_FPGA_wfmMUX.vi"("OppAux"=w433, "Aux"=w435, "Sel"=w463, "OppPri"=w421, "Pri+Aux"=w431, "OppPri+OppAux"=w426, "FGEN"=w420, "Pri+OppAux"=w427, "OppPri+Aux"=w429, "Pri"=w424) -> ("SelectedWfm"=w444:fxp<+/-,16,14>)  [unwired: 5 in]
    n372 = Multiply(x=w452, y=w450) -> (x*y=w454:fxp<+/-,48,46>)
    n373 = Multiply(x=w458, y=w456) -> (x*y=w460:fxp<+/-,48,46>)
    n374 = Multiply(x=w446, y=w444) -> (x*y=w448:fxp<+/-,48,46>)
    n375 = Scale By Power Of 2(n=i16 -30, x=w454) -> (x*2^n=w455:fxp<+/-,48,46>)
    n376 = Scale By Power Of 2(n=i16 -30, x=w460) -> (x*2^n=w459:fxp<+/-,48,46>)
    n377 = Scale By Power Of 2(n=i16 -30, x=w448) -> (x*2^n=w449:fxp<+/-,48,46>)
    n378 = To Fixed-Point(fixed-point type=w450, number=w455) -> (fixed-point=w451:fxp<+/-,16,14>)
    n379 = To Fixed-Point(fixed-point type=w456, number=w459) -> (fixed-point=w457:fxp<+/-,16,14>)
    n380 = To Fixed-Point(fixed-point type=w444, number=w449) -> (fixed-point=w445:fxp<+/-,16,14>)
    n381 = Add(x=w451, y=w475) -> (x+y=w474:fxp<+/-,16,14>)
    n382 = Add(x=w457, y=w470) -> (x+y=w469:fxp<+/-,16,14>)
    n383 = Add(x=w445, y=w465) -> (x+y=w464:fxp<+/-,16,14>)
    n384 = call "_FPGA_wfmFXPtoU14.vi"("wfmFXP"=w469) -> ("U14"=w471:fxp<+,14,14>)
    n385 = call "_FPGA_wfmFXPtoU14.vi"("wfmFXP"=w464) -> ("U14"=w466:fxp<+,14,14>)
    n386 = call "_FPGA_wfmFXPtoU14.vi"("wfmFXP"=w474) -> ("U14"=w476:fxp<+,14,14>)
    n387 = xnode ("FIFO Method Node")("Element"=w471, "Timeout"=0) -> ()  [unwired: 1 in, 2 out]
    n388 = xnode ("FIFO Method Node")("Element"=w476, "Timeout"=0) -> ()  [unwired: 1 in, 2 out]
    n389 = xnode ("FIFO Method Node")("Element"=w466, "Timeout"=0) -> ()  [unwired: 1 in, 2 out]
  }
  n390 = xnode "FPGA I/O Property Node"("FPGA I/O In"=w24, "Terminal Mode"=w23, "Voltage Range"=w22) -> ("FPGA I/O Out"=w21:refnum<k21>)
  n391 = xnode "FPGA I/O Property Node"("FPGA I/O In"=w19, "Terminal Mode"=w23, "Voltage Range"=w22) -> ("FPGA I/O Out"=w20:refnum<k21>)
  n392 = node-c288() -> (w18:T3)  [unwired: 1 in]
  n393 = timed-loop {
    timing: w18 -> [_]
    timing-out: [_] -> w17
    stop <- _ stop-if-true
    n394 = xnode ("Register Read")() -> ("Data"=w501:u16)  [unwired: 1 in, 1 out]
    n395 = xnode ("Register Read")() -> ("Data"=w512:u16)  [unwired: 1 in, 1 out]
    n396 = To Word Integer(number=w501) -> (16bit integer=w506:i16)
    n397 = feedback #69() -> (w502:bool)  [unwired: 1 in]
    n398 = call "_FPGA_Driver_FastADC.vi"("Clk_in"=w502) -> ("Clk_out"=w515:bool, "Output"=w516:i16)  [unwired: 9 in]
    n399 = call "_FPGA_Timebase.vi"("HalfPeriod"=w512) -> ("Clk_out"=w518:bool)
    n400 = Not(x=w502) -> (.not. x?=w503:bool)
    n401 = feedback-in #69(w503) -> ()
    n402 = To Long Integer(number=w516) -> (32bit integer=w514:i32)
    n403 = feedback #70() -> (w511:i16)  [unwired: 1 in]
    n404 = feedback-in #70(w506) -> ()
    n405 = feedback #71() -> (w500:i32)  [unwired: 1 in]
    n406 = feedback-in #71(w514) -> ()
    n407 = feedback #72() -> (w498:bool)  [unwired: 1 in]
    n408 = feedback-in #72(w515) -> ()
    n409 = feedback-in #73(w518) -> ()
    n410 = feedback #73() -> (w513:bool)  [unwired: 1 in]
    n411 = call <instrlib>:"Detect Rising Edge.vi"("signal"=w513) -> ("edge detected"=w495:bool)  [unwired: 14 in]
    n412 = Negate(x=w511) -> (-x=w507:i16)
    n413 = feedback #74() -> (w496:i32)  [unwired: 1 in]
    n414 = Add(x=w500, y=w496) -> (x+y=w499:i32)
    n415 = Select(t=w499, s=w498, f=w496) -> (s? t:f=w497:i32)
    n416 = Scale By Power Of 2(n=w507, x=w497) -> (x*2^n=w510:i32)
    n417 = Select(t=0 ("f"), s=w495, f=w497) -> (s? t:f=w508:i32)
    n418 = feedback-in #74(w508) -> ()
    n419 = To Word Integer(number=w510) -> (16bit integer=w504:i16)
    n420 = feedback #75() -> (w517:i16)  [unwired: 1 in]
    n421 = feedback-in #75(w504) -> ()
    n422 = feedback #76() -> (w505:bool)  [unwired: 1 in]
    n423 = feedback-in #76(w495) -> ()
    n424 = case shown="True" w505 {
      tunnel: w517 -> [_ w519]
      frame False {
      }
      frame True {
        n425 = xnode ("FIFO Method Node")("Element"=w519, "Timeout"=0) -> ()  [unwired: 1 in, 2 out]
      }
    }
  }
  n426 = while {
    tunnel: w21 -> [w524]
    tunnel: w20 -> [w523]
    stop <- FALSE stop-if-true
    n427 = xnode ("Register Read")() -> ("Data"=w525:bool)  [unwired: 1 in, 1 out]
    n428 = case shown="True" w525 {
      tunnel: [w539 w541] -> w526
      tunnel: w524 -> [_ w540]
      tunnel: w523 -> [w538 _]
      frame True {
        n429 = xnode "FPGA I/O Node"("FPGA I/O In"=w538) -> ("I/O Item"=w539:fxp<+/-,24,5>)  [unwired: 1 out]
      }
      frame False {
        n430 = xnode "FPGA I/O Node"("FPGA I/O In"=w540) -> ("I/O Item"=w541:fxp<+/-,24,5>)  [unwired: 1 out]
      }
    }
    n431 = Divide(x=w526, y=fxp<+,3,3> 5.0) -> (x/y=w529:fxp<+/-,24,1>)
    n432 = call "Tick Count"() -> ("Tick Count(Ticks)"=w535:u32)
    n433 = feedback #77() -> (w532:fxp<+/-,24,1>)  [unwired: 1 in]
    n434 = feedback-in #77(w529) -> ()
    n435 = feedback #78() -> (w536:u32)  [unwired: 1 in]
    n436 = feedback-in #78(w535) -> ()
    n437 = Multiply(x=w532, y=fxp<+,15,15> 32767.0) -> (x*y=w531:i16)
    n438 = Subtract(x=w535, y=w536) -> (x-y=→"AI.ReadingClocks":u32)
    n439 = feedback #79() -> (w527:i16)  [unwired: 1 in]
    n440 = feedback-in #79(w531) -> ()
    n441 = xnode ("FIFO Method Node")("Element"=w527, "Timeout"=-1) -> ()  [unwired: 1 in, 2 out]
  }
  n442 = while {
    stop <- FALSE stop-if-true
    n443 = xnode ("Register Read")() -> ("Data"=w543:fxp<+/-,20,5>)  [unwired: 1 in, 1 out]
    n444 = xnode ("Register Read")() -> ("Data"=w548:u32)  [unwired: 1 in, 1 out]
    n445 = xnode ("Register Read")() -> ("Data"=w545:bool)  [unwired: 1 in, 1 out]
    n446 = Number To Boolean Array(number=w548) -> (Boolean array=w547:bool[])
    n447 = Boolean Array To Number(Boolean array=w547) -> (number=w546:fxp<+/-,32,5>)
    n448 = To Fixed-Point(number=w546) -> (fixed-point=w549:fxp<+/-,20,5>)  [unwired: 1 in]
    n449 = Select(t=w543, s=w545, f=w549) -> (s? t:f=w544:fxp<+/-,20,5>)
    n450 = xnode "FPGA I/O Node"("AO2"=w544) -> ()  [unwired: 1 in, 1 out]
  }
  n451 = while {
    stop <- FALSE stop-if-true
    n452 = xnode ("Register Read")() -> ("Data"=w551:fxp<+/-,20,5>)  [unwired: 1 in, 1 out]
    n453 = xnode ("Register Read")() -> ("Data"=w556:u32)  [unwired: 1 in, 1 out]
    n454 = xnode ("Register Read")() -> ("Data"=w553:bool)  [unwired: 1 in, 1 out]
    n455 = Number To Boolean Array(number=w556) -> (Boolean array=w554:bool[])
    n456 = Boolean Array To Number(Boolean array=w554) -> (number=w555:fxp<+/-,32,5>)
    n457 = To Fixed-Point(number=w555) -> (fixed-point=w557:fxp<+/-,20,5>)  [unwired: 1 in]
    n458 = Select(t=w551, s=w553, f=w557) -> (s? t:f=w552:fxp<+/-,20,5>)
    n459 = xnode "FPGA I/O Node"("AO3"=w552) -> ()  [unwired: 1 in, 1 out]
  }
  n460 = node-c288(w17) -> ()
  n461 = node-c288(w33) -> ()
  n462 = node-c288() -> (w16:T3)  [unwired: 1 in]
  n463 = node-c288() -> (w14:T3)  [unwired: 1 in]
  n464 = node-c288() -> (w12:T3)  [unwired: 1 in]
  n465 = node-c288() -> (w30:T3)  [unwired: 1 in]
  n466 = node-c288() -> (w26:T3)  [unwired: 1 in]
  n467 = node-c288() -> (w28:T3)  [unwired: 1 in]
  n468 = node-c288() -> (w6:T3)  [unwired: 1 in]
  n469 = node-c288() -> (w4:T3)  [unwired: 1 in]
  n470 = timed-loop {
    timing: w16 -> [_]
    timing-out: [_] -> w15
    stop <- _ stop-if-true
    w570 = 0 ("Timeout")
    n471 = xnode ("FIFO Method Node")("Timeout"=w570) -> ("Element"=w571:i16, "Timed Out?"=w572:bool)  [unwired: 1 in, 1 out]
    n472 = xnode ("FIFO Method Node")("Timeout"=w570) -> ("Element"=w574:i16, "Timed Out?"=w573:bool)  [unwired: 1 in, 1 out]
    n473 = xnode ("Register Read")() -> ("Data"=w575:bool)  [unwired: 1 in, 1 out]
    n474 = case shown="True" w575 {
      tunnel: w574 -> [_ w586]
      tunnel: w573 -> [_ w585]
      tunnel: w572 -> [w583 _]
      tunnel: w571 -> [w584 _]
      tunnel: [w584 w586] -> w563
      tunnel: [w583 w585] -> w566
      frame False {
      }
      frame True {
      }
    }
    n475 = Not(x=w566) -> (.not. x?=w559:bool)
    n476 = feedback #80() -> (w568:i16)  [unwired: 1 in]
    n477 = feedback-in #80(w563) -> ()
    n478 = feedback-in #81(w559) -> ()
    n479 = feedback #81() -> (w567:bool)  [unwired: 1 in]
    n480 = xnode ("FIFO Method Node")("Timeout"=0) -> ("Element"=w561:bool, "Timed Out?"=w558:bool)  [unwired: 1 in, 1 out]
    n481 = Compound Arithmetic op=AND(w561, invert w558) -> (w560:bool)
    n482 = xnode ("Register Read")() -> ("Data"=w578:u32)  [unwired: 1 in, 1 out]
    n483 = feedback #82() -> (w564:u32)  [unwired: 1 in]
    "Daq.Length?" <- w564
    n484 = Select(t=w578, s=w560, f=w564) -> (s? t:f=w576:u32)
    n485 = feedback-in #82(w576) -> ()
    n486 = feedback #83() -> (w565:u32)  [unwired: 1 in]
    "Daq.AqNumber?" <- w565
    n487 = Select(t=u32 0, s=w560, f=w565) -> (s? t:f=w582:u32)
    n488 = Less?(x=w582, y=w576) -> (x < y?=w579:bool)
    n489 = And(x=w579, y=w567) -> (x .and. y?=w569:bool)
    n490 = xnode ("Register Write")("Data"=w579) -> ()  [unwired: 1 in, 1 out]
    n491 = call "_FPGA_HighestValueAbsI16.vi"("Enable"=w569, "Init"=w560, "Value in"=w568) -> ("Highest Value"=w580:i16)  [unwired: 8 in]
    "Daq.HighestValue_I16" <- w580
    n492 = case shown="True" w569 {
      tunnel: [w587 w590] -> w577
      tunnel: w582 -> [w587 w591]
      tunnel: w568 -> [_ w589]
      frame False {
      }
      frame True {
        n493 = xnode ("FIFO Method Node")("Element"=w589, "Timeout"=0) -> ()  [unwired: 1 in, 2 out]
        n494 = Increment(x=w591) -> (x+1=w590:u32)
      }
    }
    n495 = feedback-in #83(w577) -> ()
    n496 = xnode ("Register Write")("Data"=w580) -> ()  [unwired: 1 in, 1 out]
  }
  n497 = timed-loop {
    timing: w14 -> [_]
    timing-out: [_] -> w13
    stop <- _ stop-if-true
    n498 = xnode ("Register Read")() -> ("Data"=w596:u8)  [unwired: 1 in, 1 out]
    n499 = case shown="4" w596 {
      tunnel: [w597 w598 w599 w600 w601] -> w595
      frame 0, Default {
        n500 = xnode ("Register Read")() -> ("Data"=w597:bool)  [unwired: 1 in, 1 out]
      }
      frame 1 {
        n501 = xnode ("Register Read")() -> ("Data"=w598:bool)  [unwired: 1 in, 1 out]
      }
      frame 3 {
        n502 = xnode ("Register Read")() -> ("Data"=w599:bool)  [unwired: 1 in, 1 out]
      }
      frame 4 {
        n503 = xnode ("Register Write")() -> ("Data"=w600:bool)  [unwired: 1 in, 1 out]
      }
      frame 2 {
        n504 = xnode ("Register Read")() -> ("Data"=w601:bool)  [unwired: 1 in, 1 out]
      }
    }
    n505 = feedback-in #84(w595) -> ()
    n506 = feedback #84() -> (w594:bool)  [unwired: 1 in]
    n507 = xnode "DO0"("DIO0"=w594) -> ()  [unwired: 1 in, 1 out]
  }
  n508 = timed-loop {
    timing: w12 -> [_]
    timing-out: [_] -> w11
    stop <- _ stop-if-true
    n509 = xnode ("Register Read")() -> ("Data"=w606:u8)  [unwired: 1 in, 1 out]
    n510 = case shown="4" w606 {
      tunnel: [w607 w608 w609 w610 w611] -> w605
      frame 0, Default {
        n511 = xnode ("Register Read")() -> ("Data"=w607:bool)  [unwired: 1 in, 1 out]
      }
      frame 1 {
        n512 = xnode ("Register Read")() -> ("Data"=w608:bool)  [unwired: 1 in, 1 out]
      }
      frame 2 {
        n513 = xnode ("Register Read")() -> ("Data"=w609:bool)  [unwired: 1 in, 1 out]
      }
      frame 3 {
        n514 = xnode ("Register Read")() -> ("Data"=w610:bool)  [unwired: 1 in, 1 out]
      }
      frame 4 {
        n515 = xnode ("Register Write")() -> ("Data"=w611:bool)  [unwired: 1 in, 1 out]
      }
    }
    n516 = feedback-in #85(w605) -> ()
    n517 = feedback #85() -> (w604:bool)  [unwired: 1 in]
    n518 = xnode "DO1"("DIO1"=w604) -> ()  [unwired: 1 in, 1 out]
  }
  n519 = timed-loop {
    timing: w30 -> [_]
    timing-out: [_] -> w29
    stop <- _ stop-if-true
    n520 = xnode ("FIFO Method Node")("Timeout"=0) -> ("Element"=w615:fxp<+,14,14>, "Timed Out?"=w616:bool)  [unwired: 1 in, 1 out]
    n521 = Not(x=w616) -> (.not. x?=w617:bool)
    n522 = feedback #86() -> (w618:bool)  [unwired: 1 in]
    n523 = Not(x=w618) -> (.not. x?=w619:bool)
    n524 = feedback-in #86(w619) -> ()
    n525 = feedback #87() -> (w614:fxp<+,14,14>)  [unwired: 1 in]
    n526 = feedback-in #87(w615, w617) -> ()
    n527 = call "_FPGA_Driver_LTC1667_1_v1_3.vi"("Clk"=w618, "Data in"=w614) -> ()  [unwired: 10 in]
  }
  n528 = timed-loop {
    timing: w26 -> [_]
    timing-out: [_] -> w25
    stop <- _ stop-if-true
    n529 = xnode ("FIFO Method Node")("Timeout"=0) -> ("Element"=w624:fxp<+,14,14>, "Timed Out?"=w625:bool)  [unwired: 1 in, 1 out]
    n530 = Not(x=w625) -> (.not. x?=w626:bool)
    n531 = feedback #88() -> (w628:bool)  [unwired: 1 in]
    n532 = Not(x=w628) -> (.not. x?=w629:bool)
    n533 = feedback-in #88(w629) -> ()
    n534 = feedback #89() -> (w623:fxp<+,14,14>)  [unwired: 1 in]
    n535 = feedback-in #89(w624, w626) -> ()
    n536 = call "_FPGA_Driver_LTC1667_2_v1_3.vi"("Clk"=w628, "Data in"=w623) -> ()  [unwired: 10 in]
  }
  n537 = timed-loop {
    timing: w28 -> [_]
    timing-out: [_] -> w27
    stop <- _ stop-if-true
    n538 = xnode ("FIFO Method Node")("Timeout"=0) -> ("Element"=w634:fxp<+,14,14>, "Timed Out?"=w636:bool)  [unwired: 1 in, 1 out]
    n539 = Not(x=w636) -> (.not. x?=w635:bool)
    n540 = feedback #90() -> (w637:bool)  [unwired: 1 in]
    n541 = Not(x=w637) -> (.not. x?=w638:bool)
    n542 = feedback-in #90(w638) -> ()
    n543 = feedback-in #91(w634, w635) -> ()
    n544 = feedback #91() -> (w633:fxp<+,14,14>)  [unwired: 1 in]
    n545 = call "_FPGA_Driver_LTC1667_3_v1.3.vi"("Clk"=w637, "Data_in"=w633) -> ()  [unwired: 10 in]
  }
  n546 = timed-loop {
    timing: w6 -> [_]
    timing-out: [_] -> w5
    stop <- _ stop-if-true
    n547 = xnode ("Register Read")() -> ("Data"=w643:u8)  [unwired: 1 in, 1 out]
    n548 = call "_FPGA_Driver_V1.4DIO.vi"("DO"=w643) -> ("DI"=w642:u8)  [unwired: 10 in]
    n549 = xnode ("Register Write")("Data"=w642) -> ()  [unwired: 1 in, 1 out]
    n550 = feedback-in #92(w642) -> ()
    n551 = feedback #92() -> (→"DI":u8)  [unwired: 1 in]
  }
  n552 = timed-loop "AO (AD5648)" {
    timing: w4 -> [_]
    timing-out: [_] -> w3
    stop <- _ stop-if-true
    n553 = xnode ("Register Read")() -> ("Data"=w648:u8)  [unwired: 1 in, 1 out]
    n554 = xnode ("Register Read")() -> ("Data"=w649:bool)  [unwired: 1 in, 1 out]
    n555 = xnode ("Register Read")() -> ("Data"=w646:u8)  [unwired: 1 in, 1 out]
    n556 = xnode ("Register Read")() -> ("Data"=w647:u16)  [unwired: 1 in, 1 out]
    n557 = call "_FPGA_Driver_AD5648_v1.4.vi"("Cmd#"=w646, "AO Data"=w647, "Channel#"=w648, "Update_latch"=w649) -> ("Updating?"=w650:bool)  [unwired: 7 in]
    n558 = xnode ("Register Write")("Data"=w650) -> ()  [unwired: 1 in, 1 out]
  }
  n559 = node-c288(w29) -> ()
  n560 = node-c288(w25) -> ()
  n561 = node-c288(w27) -> ()
  n562 = node-c288(w5) -> ()
  n563 = node-c288(w3) -> ()
  n564 = node-c288(w13) -> ()
  n565 = node-c288(w11) -> ()
  n566 = node-c288() -> (w10:T3)  [unwired: 1 in]
  n567 = node-c288() -> (w8:T3)  [unwired: 1 in]
  n568 = timed-loop {
    timing: w10 -> [_]
    timing-out: [_] -> w9
    stop <- _ stop-if-true
    n569 = xnode ("Register Read")() -> ("Data"=w655:u8)  [unwired: 1 in, 1 out]
    n570 = case shown="4" w655 {
      tunnel: [w656 w657 w658 w659 w660] -> w654
      frame 0, Default {
        n571 = xnode ("Register Read")() -> ("Data"=w656:bool)  [unwired: 1 in, 1 out]
      }
      frame 1 {
        n572 = xnode ("Register Read")() -> ("Data"=w657:bool)  [unwired: 1 in, 1 out]
      }
      frame 2 {
        n573 = xnode ("Register Read")() -> ("Data"=w658:bool)  [unwired: 1 in, 1 out]
      }
      frame 3 {
        n574 = xnode ("Register Read")() -> ("Data"=w659:bool)  [unwired: 1 in, 1 out]
      }
      frame 4 {
        n575 = xnode ("Register Write")() -> ("Data"=w660:bool)  [unwired: 1 in, 1 out]
      }
    }
    n576 = feedback-in #93(w654) -> ()
    n577 = feedback #93() -> (w653:bool)  [unwired: 1 in]
    n578 = xnode "DO2"("DIO2"=w653) -> ()  [unwired: 1 in, 1 out]
  }
  n579 = timed-loop {
    timing: w8 -> [_]
    timing-out: [_] -> w7
    stop <- _ stop-if-true
    n580 = xnode ("Register Read")() -> ("Data"=w664:u8)  [unwired: 1 in, 1 out]
    n581 = case shown="4" w664 {
      tunnel: [w666 w667 w668 w669 w670] -> w665
      frame 0, Default {
        n582 = xnode ("Register Read")() -> ("Data"=w666:bool)  [unwired: 1 in, 1 out]
      }
      frame 1 {
        n583 = xnode ("Register Read")() -> ("Data"=w667:bool)  [unwired: 1 in, 1 out]
      }
      frame 2 {
        n584 = xnode ("Register Read")() -> ("Data"=w668:bool)  [unwired: 1 in, 1 out]
      }
      frame 3 {
        n585 = xnode ("Register Read")() -> ("Data"=w669:bool)  [unwired: 1 in, 1 out]
      }
      frame 4 {
        n586 = xnode ("Register Write")() -> ("Data"=w670:bool)  [unwired: 1 in, 1 out]
      }
    }
    n587 = feedback-in #94(w665) -> ()
    n588 = feedback #94() -> (w663:bool)  [unwired: 1 in]
    n589 = xnode "DO3"("DIO3"=w663) -> ()  [unwired: 1 in, 1 out]
  }
  n590 = node-c288(w9) -> ()
  n591 = node-c288(w7) -> ()
  n592 = node-c288(w15) -> ()
